vi "Get dBm Impedance.vi"(8 "error in (no error)":errorcluster, 11 "VISA resource name":refnum<visa-resource-name>) -> (0 "error out":errorcluster, 2 "dBm Impedance":i32, 3 "VISA resource name out":refnum<visa-resource-name>)   [LabVIEW 2011, in "Fluke 5XXX Series Multicalibrators.lvlib"]
doc: "This VI gets the impedance used for dBm outputs (ac volts).\n\nNote:\n\nThis VI is available only for instrument model 5520A."
uses:
  Fluke 5XXX Series Multicalibrators.lvlib
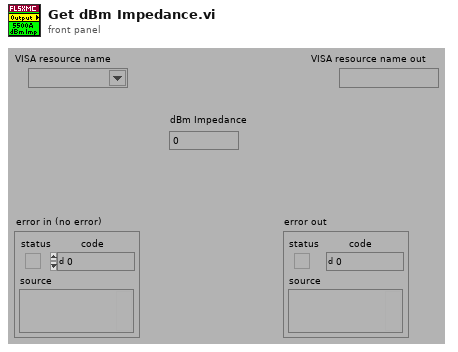
[diagram p1: front panel]
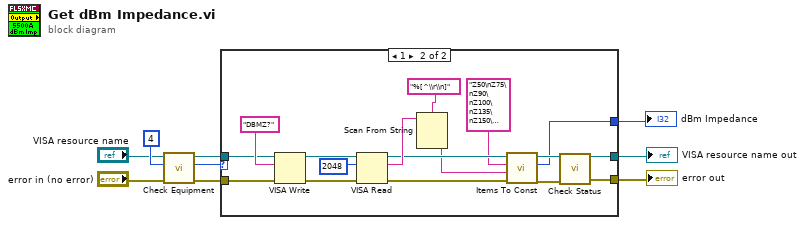
[diagram p0: block diagram]
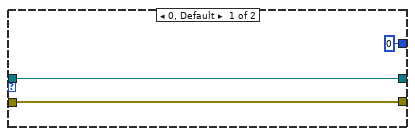
[diagram p2: hidden frame]
diagram:
  n1 = call "Check Equipment.vi"("error in (no error)"="error in (no error)", "Bit Mask"=4 ("Numeric"), "VISA resource name"="VISA resource name") -> ("error out"=w8:errorcluster, "Present?"=w7:u32, "VISA resource name out"=w6:refnum<visa-resource-name>)  [unwired: 6 in]
  n2 = case shown="1" w7 {
    tunnel: [w11 w21] -> w2
    tunnel: w8 -> [w12 w23]
    tunnel: w6 -> [w11 w22]
    tunnel: [w12 w20] -> w5
    tunnel: [0 ("Index") w15] -> w1
    frame 0, Default {
    }
    frame 1 {
      n3 = VISA Write(VISA resource name=w22, write buffer="DBMZ?", error in (no error)=w23) -> (VISA resource name out=w28:refnum<visa-resource-name>, error out=w27:errorcluster)  [unwired: 1 out]
      n4 = VISA Read(VISA resource name=w28, byte count=u32 2048 ("byte count (0)"), error in (no error)=w27) -> (VISA resource name out=w17:refnum<visa-resource-name>, read buffer=w24:string, error out=w18:errorcluster)  [unwired: 1 out]
      n5 = Scan From String(format string="%[^\\r\\n]", input string=w24) -> (output 1=w13:string)  [unwired: 3 in, 3 out]
      n6 = call "Items To Const.vi"("error in (no error)"=w18, "String Item"=w13, "Multi-Line String"="Z50\nZ75\nZ90\nZ100\nZ135\nZ150\nZ300\nZ600\nZ900\nZ1000\nZ1200", "VISA resource name"=w17) -> ("error out"=w19:errorcluster, "Index"=w15:i32, "VISA resource name out"=w16:refnum<visa-resource-name>)  [unwired: 5 in]
      n7 = call "Check Status.vi"("VISA resource name"=w16, "error in (no error)"=w19) -> ("VISA resource name out"=w21:refnum<visa-resource-name>, "error out"=w20:errorcluster)  [unwired: 12 in]
    }
  }
  "dBm Impedance" <- w1
  "VISA resource name out" <- w2
  "error out" <- w5
